vi "CRYGet Message VI Name.vi"() -> (1 "Return Flag":bool, 3 "VI Name Out":string caption="aa")   [LabVIEW 2013]
panel:
  in  "VI Name":string caption="aa"
  out "Comment":string caption="False_Comment"
  in  "Cancel":bool
  in  "OK":bool
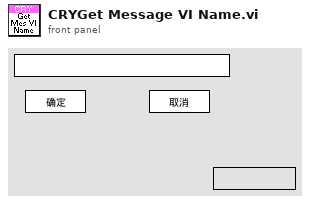
[diagram p1: front panel]
types:
  T1 = enum16{"OK", "Yes", "YesNo", "YesNoCancel", "ReplaceAppend"}
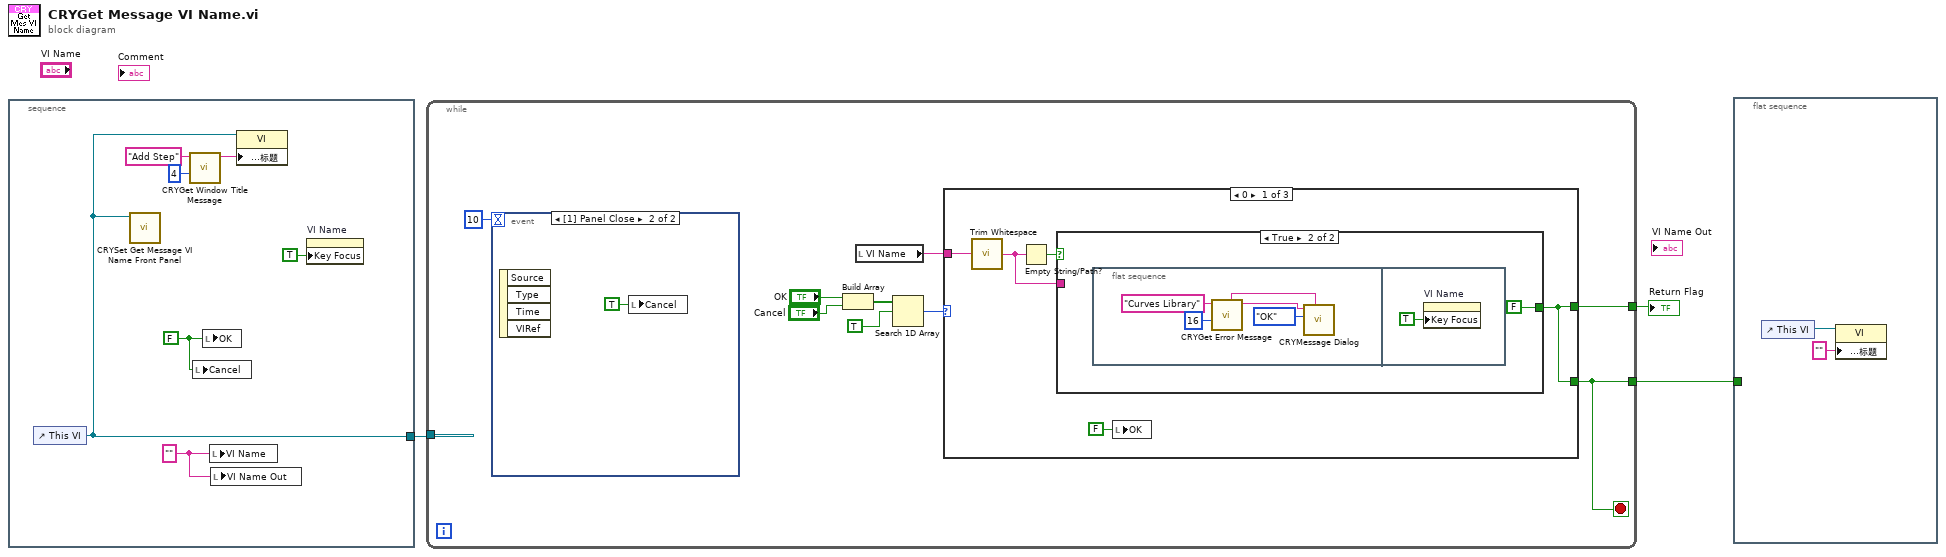
[diagram p0: block diagram]
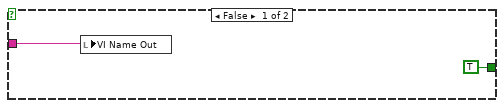
[diagram p2: hidden frame]
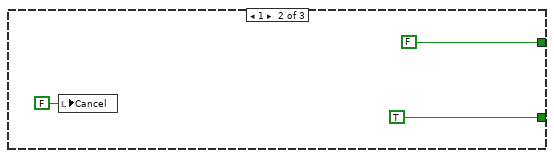
[diagram p3: hidden frame]
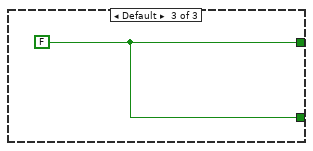
[diagram p4: hidden frame]
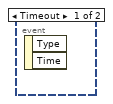
[diagram p5: hidden frame]
diagram:
  n1 = stacked-sequence {
    tunnel: [w6] -> w2
    frame #0 {
      w5 = "" ("VI Name")
      w10 = FALSE ("Yes")
      n2 = control-ref of="This VI"() -> (w6:refnum<vi>)
      n3 = call "CRYSet Get Message VI Name Front Panel.vi"("Vi Ref"=w6) -> ()  [unwired: 11 in]
      n4 = call "CRYGet Window Title Message.vi"("No"=4, "Kind"="Add Step") -> ("Multibyte String"=w7:string)  [unwired: 4 in, 5 out]
      n5 = local write "Cancel"(w10) -> ()
      n6 = local write "OK"(w10) -> ()
      n7 = local write "VI Name"(w5) -> ()
      n8 = local write "VI Name Out"(w5) -> ()
      n9 = property class="VI"(reference=w6, "前面板窗口:标题"=w7) -> ()  [unwired: 1 in, 2 out]
      n10 = property on="VI Name" class="Str"("Key Focus"=TRUE) -> ()  [unwired: 2 in, 2 out]
    }
  }
  n11 = while {
    tunnel: w2 -> [_]
    tunnel: [w12] -> w3
    tunnel: [w11] -> w1
    stop <- w11 stop-if-true
    n12 = event shown="[1] Panel Close" {
      selector: _ -> [_ _]
      dyn-events: _ -> [_ _]
      timeout: 10 -> [_ _]
      event Timeout {
        n13 = event-data() -> ()  [unwired: 1 in, 2 out]
      }
      event Panel Close {
        n14 = event-data() -> ()  [unwired: 1 in, 4 out]
        n15 = local write "Cancel"(TRUE ("Cancel")) -> ()
      }
    }
    n16 = Build Array("OK", "Cancel") -> (w15:bool[])
    n17 = local read "VI Name"() -> (w13:string)
    n18 = Search 1D Array(1D array=w15, element=TRUE) -> (index of element=w14:i32)  [unwired: 1 out]
    n19 = case shown="0" w14 {
      tunnel: w13 -> [w24 _ _]
      tunnel: [w20 FALSE ("element") w37] -> w12
      tunnel: [w20 TRUE ("element") w37] -> w11
      frame 0 {
        n20 = call <vilib>:"Trim Whitespace.vi"("string"=w24) -> ("trimmed string"=w22:string)  [unwired: 1 in]
        n21 = Empty String/Path?(string/path=w22) -> (empty?=w23:bool)
        n22 = case shown="True" w23 {
          tunnel: w22 -> [w25 _]
          tunnel: [TRUE ("element") FALSE ("element")] -> w20
          frame False {
            n23 = local write "VI Name Out"(w25) -> ()
          }
          frame True {
            n24 = flat-sequence {
              frame #0 {
                n25 = call "CRYGet Error Message.vi"("Error No"=16, "Kind"="Curves Library") -> ("Message"=w31:string, "Window Title"=w32:string)  [unwired: 4 in, 4 out]
                n26 = call "CRYMessage Dialog.vi"("Window Title"=w32, "YesNoCancel"=T1."OK", "Message Content"=w31) -> ()  [unwired: 7 in, 2 out]
              }
              frame #1 {
                n27 = property on="VI Name" class="Str"("Key Focus"=TRUE) -> ()  [unwired: 2 in, 2 out]
              }
            }
          }
        }
        n28 = local write "OK"(FALSE ("OK")) -> ()
      }
      frame 1 {
        n29 = local write "Cancel"(FALSE ("Cancel")) -> ()
      }
      frame Default {
        w37 = FALSE ("element")
      }
    }
  }
  "Return Flag" <- w3
  n30 = flat-sequence {
    tunnel: w1 -> [_]
    frame #0 {
      n31 = control-ref of="This VI"() -> (w39:refnum<vi>)
      n32 = property class="VI"(reference=w39, "前面板窗口:标题"="" ("Front Panel Window:Title")) -> ()  [unwired: 1 in, 2 out]
    }
  }
